vi "读保持寄存器.vi"(7 "MB_实体":refnum<class "Modbus Master.lvclass">, 8 "error in":errorcluster, 11 "读保持寄存器信息组__输入":T1(array[cluster])) -> (0 "输出簇":errorcluster, 3 "读保持寄存器信息组_输出":T1(array[cluster]), 5 "连接成功":bool)   [LabVIEW 2020]
uses:
  <vilib>/NI/Modbus Library/API/Master/Modbus Master.lvclass
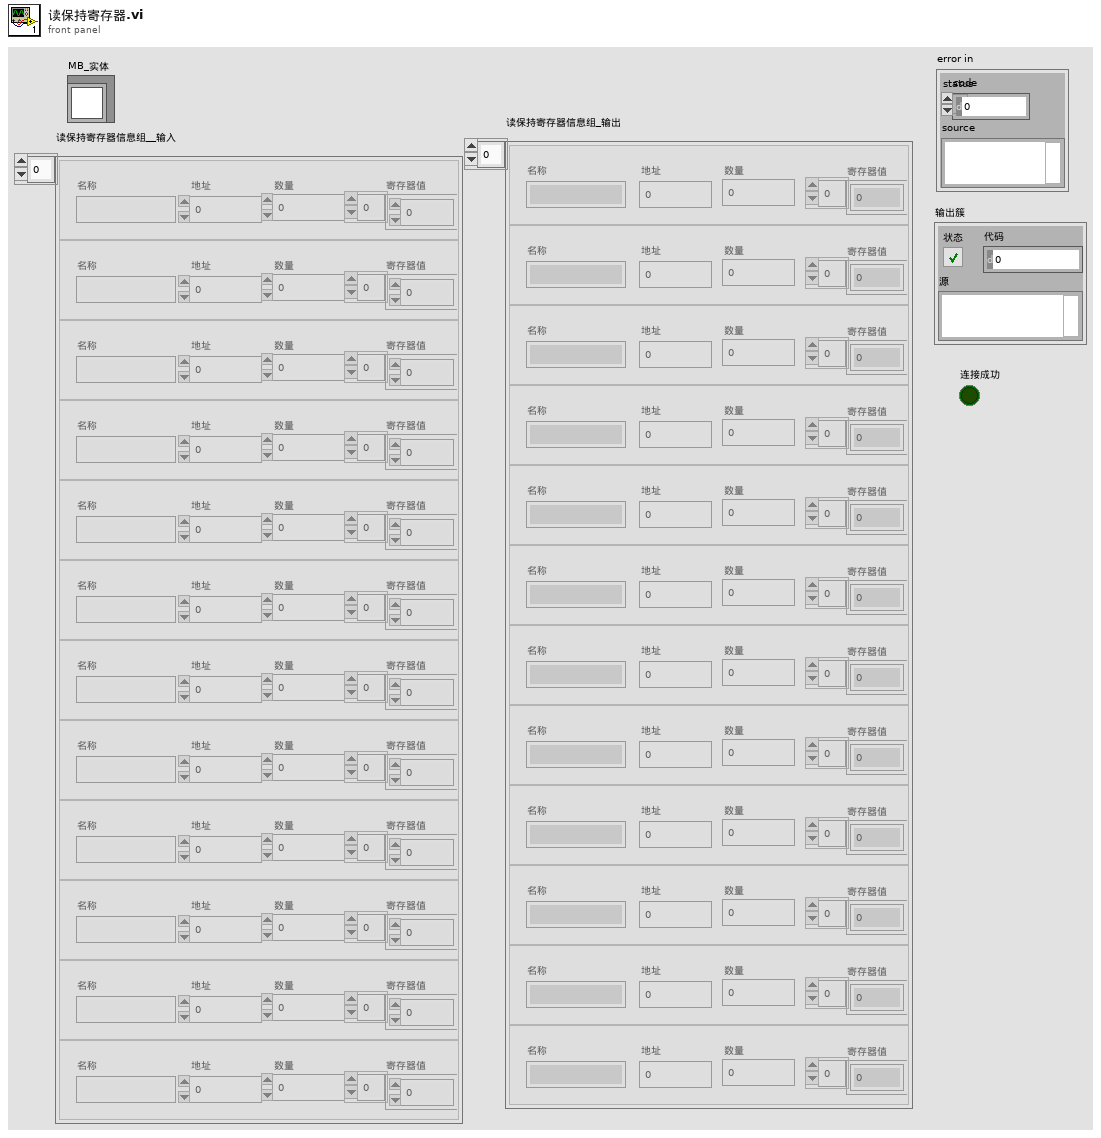
[diagram p1: front panel]
types:
  T1 = cluster{"地址":u16, "数量":u16, "寄存器值":u16[], "名称":string}[]
  T2 = cluster{"地址":u16, "数量":u16, "寄存器值":u16[], "名称":string}
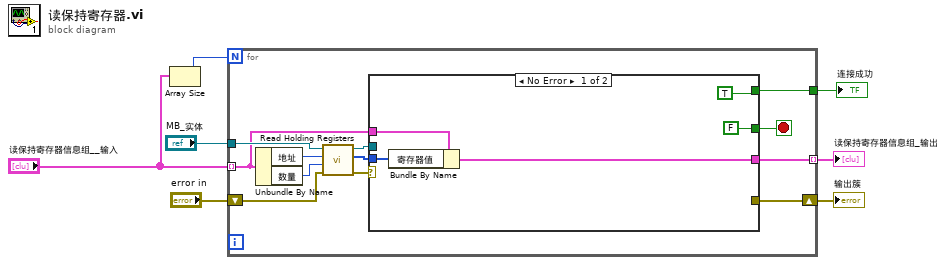
[diagram p0: block diagram]
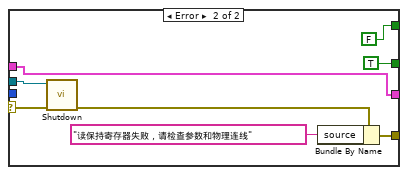
[diagram p2: hidden frame]
diagram:
  n1 = Array Size(array="读保持寄存器信息组__输入") -> (size(s)=w4:i32)
  n2 = for {
    N: w4 -> [_]
    tunnel: "读保持寄存器信息组__输入" -> [w13] mode=indexing
    tunnel: [w11] -> w7 mode=indexing
    tunnel: "MB_实体" -> [w14]
    shift-right: [w9] -> w2
    shift-left: "error in" -> [w10]
    tunnel: [w8] -> w1
    stop <- w16 stop-if-true
    n3 = Unbundle By Name(w13) -> ("地址"=w18:u16, "数量"=w17:u16)
    n4 = call-dynamic "Read Holding Registers.vi"("error in"=w10, "number of inputs"=w17, "starting address"=w18, "Modbus master in"=w14) -> ("error out"=w19:errorcluster, "register values"=w12:u16[], "Modbus master out"=w15:refnum<class "Modbus Master.lvclass">)  [unwired: 5 in]
    n5 = case shown="No Error" w19 {
      selector: w19 -> [_ w30]
      tunnel: w15 -> [_ w29]
      tunnel: [FALSE TRUE] -> w16
      tunnel: w13 -> [w23 w31]
      tunnel: w12 -> [w22 _]
      tunnel: [w21 w31] -> w11
      tunnel: [_ w27] -> w9
      tunnel: [TRUE FALSE] -> w8
      frame No Error {
        n6 = Bundle By Name(cluster=w23, "寄存器值"=w22) -> (w21:T2)
      }
      frame Error {
        n7 = call-dynamic "Shutdown.vi"("error in"=w30, "Modbus master in"=w29) -> ("error out"=w28:errorcluster)  [unwired: 9 in]
        n8 = Bundle By Name(cluster=w28, "source"="读保持寄存器失败，请检查参数和物理连线" ("消息")) -> (w27:errorcluster)
      }
    }
  }
  "读保持寄存器信息组_输出" <- w7
  "输出簇" <- w2
  "连接成功" <- w1
